vi "ReadData.vi"(4 "错误输入（队列）":errorcluster caption="错误输入（无错误）", 5 "队列输入":refnum<queue>, 6 "错误输入（采集）":errorcluster caption="错误输入（无错误）", 7 "Task In":refnum<k21>) -> (0 "错误输出（队列）":errorcluster caption="error out", 1 "队列输出":refnum<queue>, 2 "错误输出（采集）":errorcluster caption="错误输出", 3 "Task Out":refnum<k21> caption="任务输出")   [LabVIEW 2012]
uses:
  <vilib>/DAQmx/read.llb/DAQmx Read (Analog 1D Wfm NChan NSamp).vi
  GlobalVariable.vi
  <vilib>/DAQmx/miscellaneous.llb/DAQmx Fill In Error Info.vi
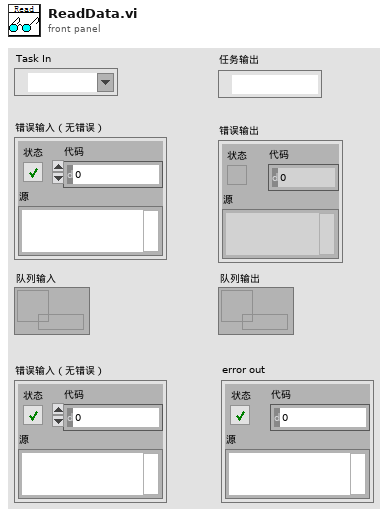
[diagram p1: front panel]
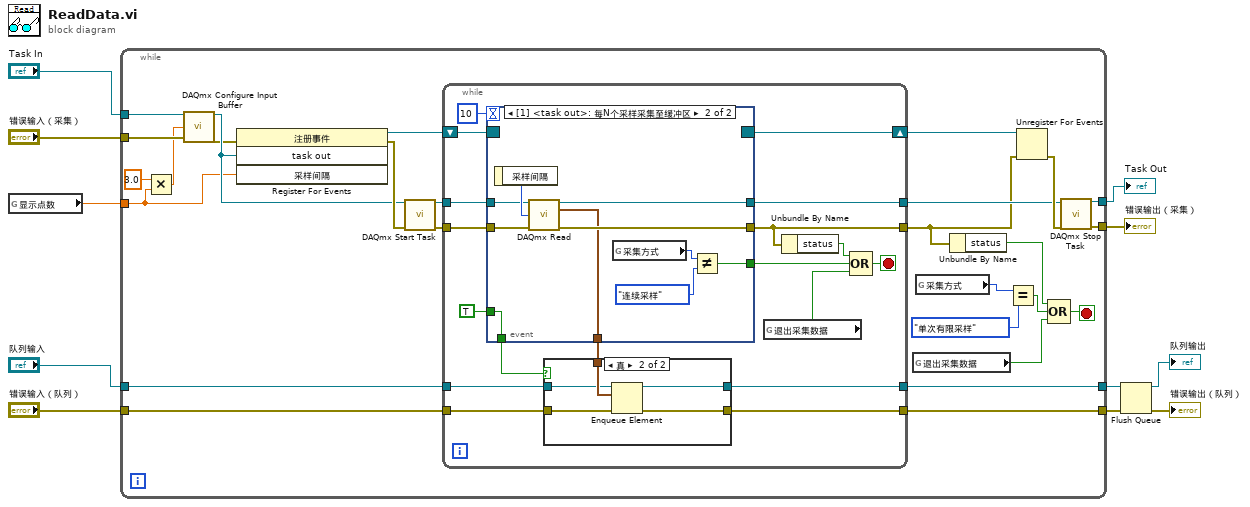
[diagram p0: block diagram]
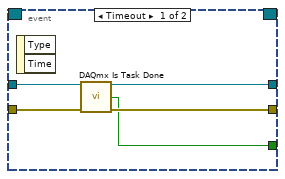
[diagram p3: hidden frame]
diagram:
  n1 = global read "GlobalVariable.vi" "显示点数"() -> (w7:dbl)
  n2 = while {
    tunnel: "错误输入（采集）" -> [w17]
    tunnel: w7 -> [w16]
    tunnel: "Task In" -> [w18]
    tunnel: [w31] -> w9
    tunnel: [w30] -> w8
    tunnel: "队列输入" -> [w22]
    tunnel: "错误输入（队列）" -> [w21]
    tunnel: [w13] -> w4
    tunnel: [w12] -> w3
    stop <- w28 stop-if-true
    n3 = Multiply(x=3.0, y=w16) -> (x*y=w14:dbl)
    n4 = call <vilib>:"DAQmx Configure Input Buffer.vi"("task/channels in"=w18, "buffer size (in samples per channel)"=w14, "error in"=w17) -> ("task out"=w20:refnum<k21>, "error out"=w19:errorcluster)  [unwired: 11 in]
    n5 = register-events(error in=w19, w20, w16) -> (reference out=w34:refnum<event-registration>, error out=w38:errorcluster)  [unwired: 1 in]
    n6 = call <vilib>:"DAQmx Start Task.vi"("task/channels in"=w20, "error in"=w38) -> ("task out"=w33:refnum<k21>, "error out"=w32:errorcluster)  [unwired: 12 in]
    n7 = while {
      tunnel: w33 -> [w53]
      tunnel: w32 -> [w52]
      tunnel: [w50] -> w26
      tunnel: [w48] -> w35
      shift-right: [w51] -> w37
      shift-left: w34 -> [w54]
      tunnel: w22 -> [w42]
      tunnel: w21 -> [w41]
      tunnel: [w40] -> w13
      tunnel: [w39] -> w12
      stop <- w49 stop-if-true
      n8 = event shown="[1] <task out>: 每N个采样采集至缓冲区" {
        selector: w54 -> [_ _]
        dyn-events: [_ _] -> w51
        timeout: 10 -> [_ _]
        tunnel: TRUE -> [_ w72]
        tunnel: w53 -> [w68 w76]
        tunnel: w52 -> [w67 w78]
        tunnel: [w66 w75] -> w48
        tunnel: [w65 w74] -> w50
        tunnel: [_ w73] -> w43
        tunnel: [_ w72] -> w44
        tunnel: [w64 w70] -> w46
        event Timeout {
          n9 = event-data() -> ()  [unwired: 1 in, 2 out]
          n10 = call <vilib>:"DAQmx Is Task Done.vi"("task/channels in"=w68, "error in"=w67) -> ("task out"=w66:refnum<k21>, "task done?"=w64:bool, "error out"=w65:errorcluster)  [unwired: 11 in]
        }
        event Every N Samples Acquired into Buffer {
          n11 = event-data() -> ("采样间隔"=w77:u32)  [unwired: 1 in]
          n12 = call-poly <vilib>:"DAQmx Read.vi"("task/channels in"=w76, "number of samples per channel"=w77, "error in"=w78) -> ("task out"=w75:refnum<k21>, "data"=w73:waveform(dbl)[], "error out"=w74:errorcluster)  [unwired: 10 in]
          n13 = global read "GlobalVariable.vi" "采集方式"() -> (w69:enum16{"单次有限采样", "多次有限采样", "连续采样"})
          n14 = Not Equal?(x=w69, y=enum16{"单次有限采样", "多次有限采样", "连续采样"}."连续采样") -> (x != y?=w70:bool)
        }
      }
      n15 = case shown="真" w44 {
        tunnel: w43 -> [_ w63]
        tunnel: w42 -> [w58 w62]
        tunnel: w41 -> [w57 w61]
        tunnel: [w58 w60] -> w40
        tunnel: [w57 w59] -> w39
        frame False {
        }
        frame True {
          n16 = Enqueue Element(queue=w62, element=w63, error in (no error)=w61) -> (queue out=w60:refnum<queue>, error out=w59:errorcluster)  [unwired: 1 in, 1 out]
        }
      }
      n17 = global read "GlobalVariable.vi" "退出采集数据"() -> (w45:bool)
      n18 = Unbundle By Name(w50) -> ("status"=w47:bool)
      n19 = Compound Arithmetic op=OR(w47, w46, w45) -> (w49:bool)
    }
    n20 = global read "GlobalVariable.vi" "退出采集数据"() -> (w24:bool)
    n21 = global read "GlobalVariable.vi" "采集方式"() -> (w23:enum16{"单次有限采样", "多次有限采样", "连续采样"})
    n22 = Unbundle By Name(w26) -> ("status"=w25:bool)
    n23 = Equal?(x=w23, y=enum16{"单次有限采样", "多次有限采样", "连续采样"}."单次有限采样") -> (x = y?=w27:bool)
    n24 = Unregister For Events(event registration refnum=w37, error in=w26) -> (error out=w36:errorcluster)
    n25 = Compound Arithmetic op=OR(w25, w27, w24) -> (w28:bool)
    n26 = call <vilib>:"DAQmx Stop Task.vi"("task/channels in"=w35, "error in"=w36) -> ("task out"=w31:refnum<k21>, "error out"=w30:errorcluster)  [unwired: 12 in]
  }
  "Task Out" <- w9
  "错误输出（采集）" <- w8
  n27 = Flush Queue(queue=w4, error in (no error)=w3) -> (queue out=→"队列输出":refnum<queue>, error out=→"错误输出（队列）":errorcluster)  [unwired: 1 out]
